vi "Update Crash Log.vi"(8 "New Crash Log Data":T1, 11 "Old Crash Log Data":T1) -> (3 "Updated Crash Log Data":T1)   [LabVIEW 2018, in "File IO.lvlib"]
doc: "Remove old data and add new data to the crash log."
uses:
  File IO.lvlib
  Top Level/Shared Controls/Analyzed Data Sets.ctl
  Top Level/Shared Controls/All Data Cluster.ctl
  Top Level/Shared Controls/Acq Data.ctl
  Top Level/Shared Controls/Post-Analysis Data.ctl
  Top Level/Shared Controls/Calculated Data.ctl
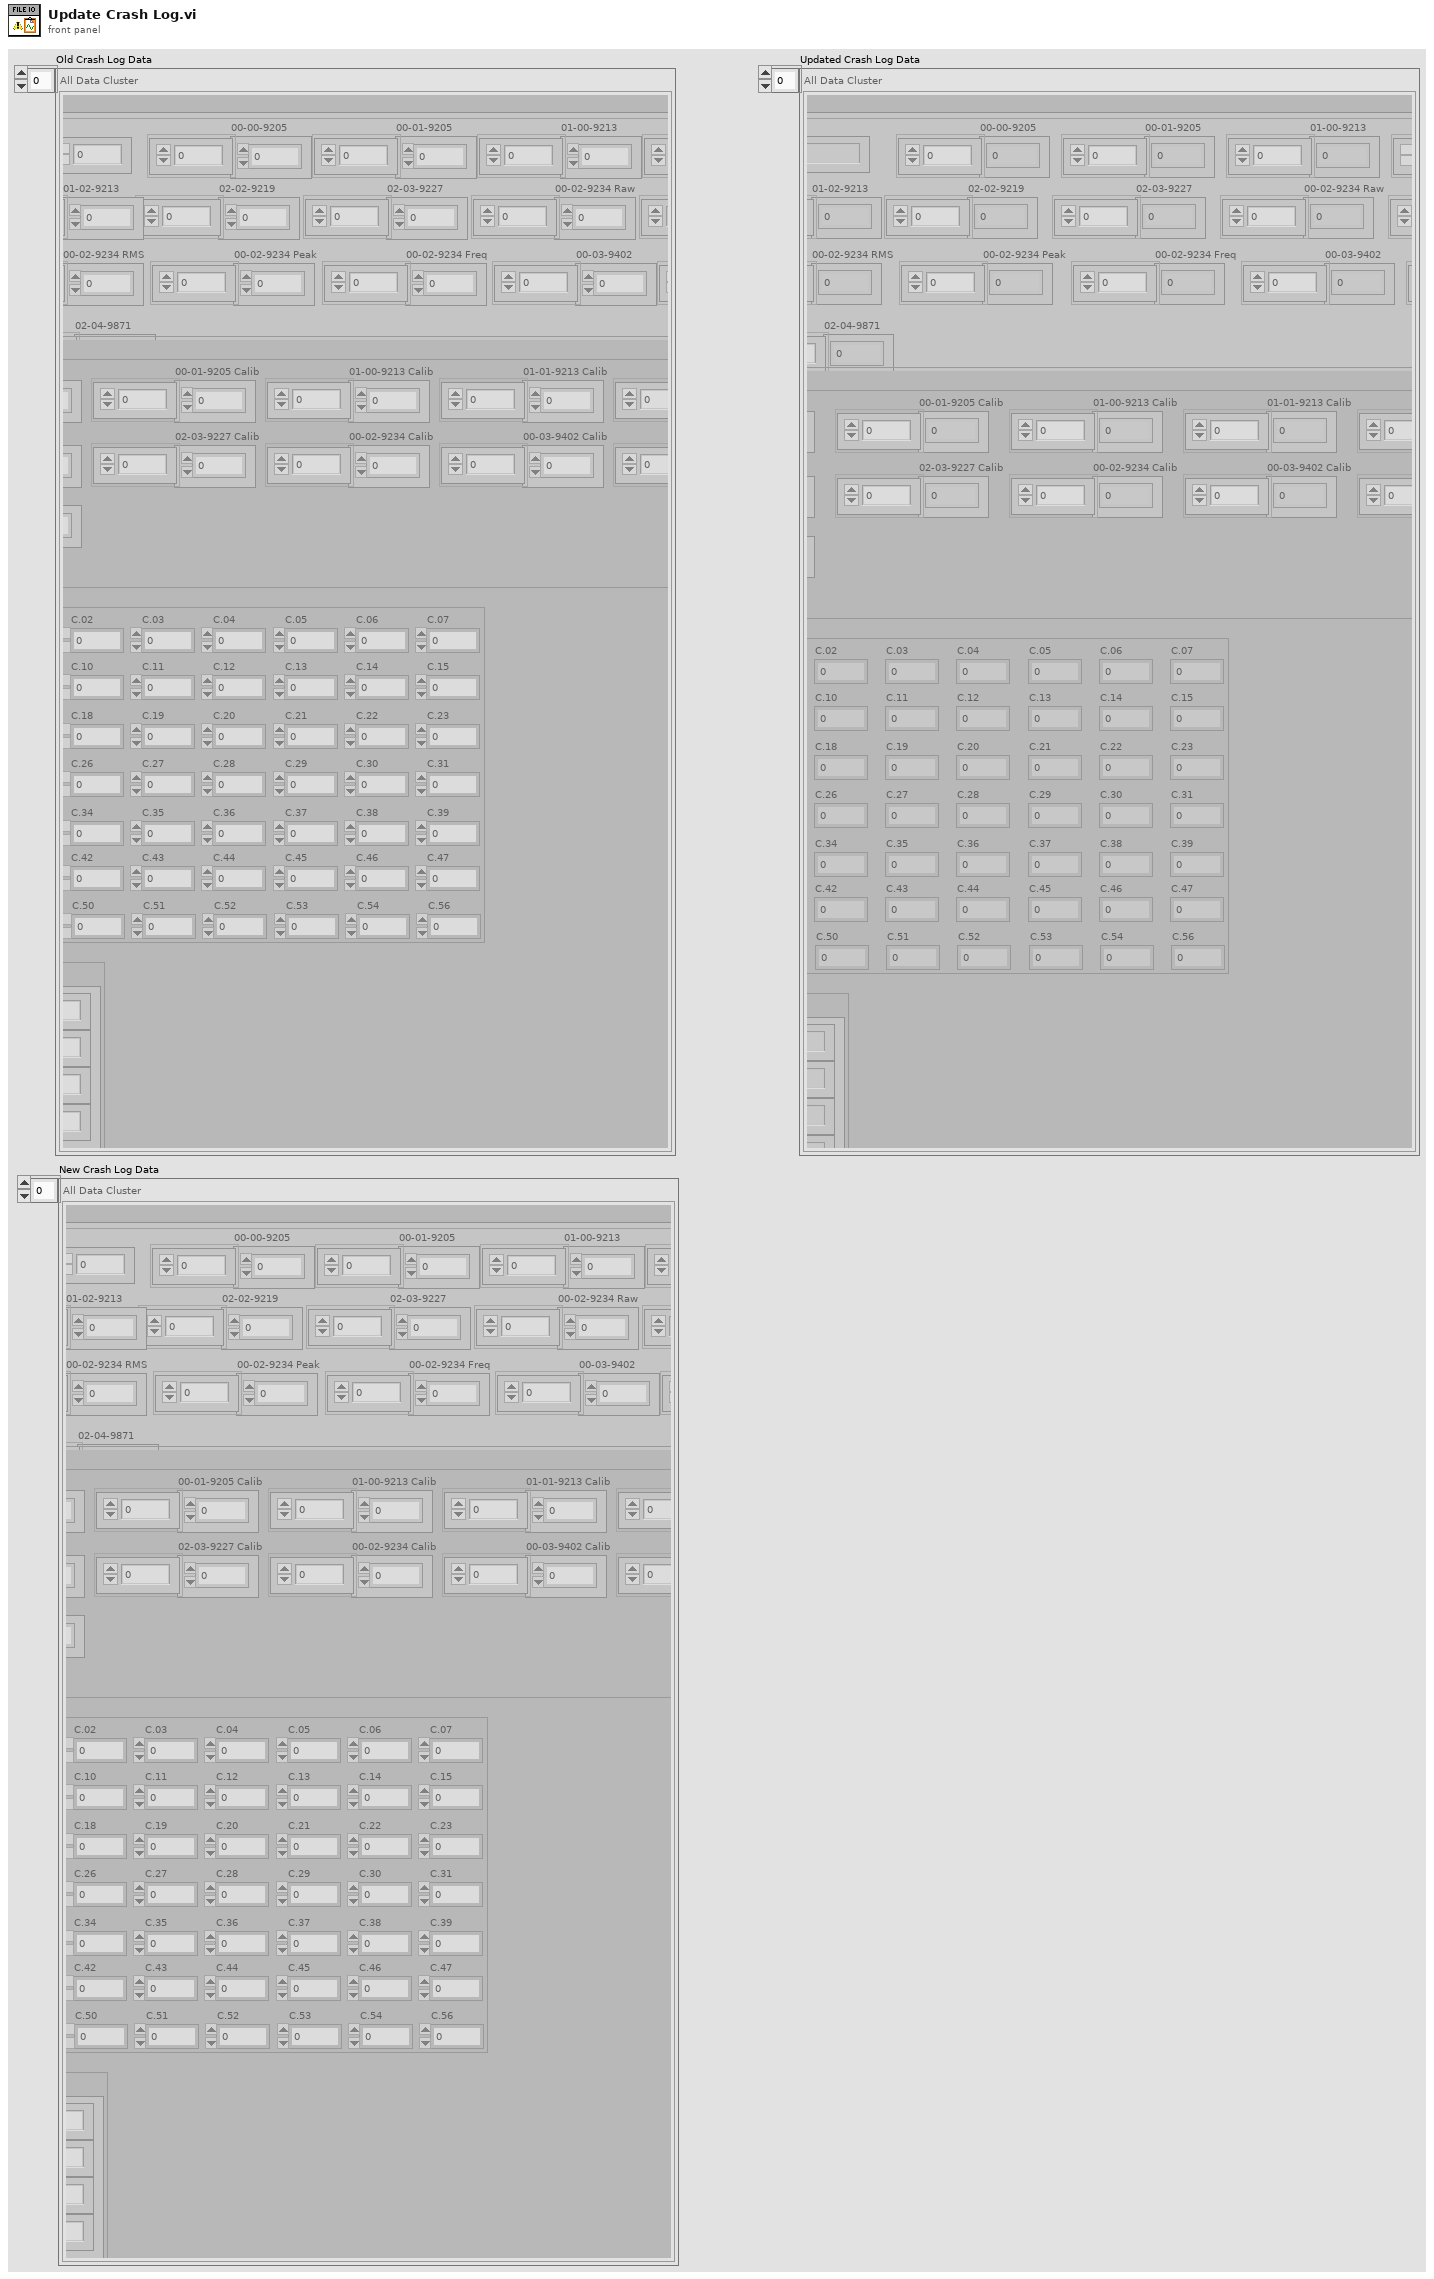
[diagram p1: front panel]
types:
  T1 = typedef "Analyzed Data Sets.ctl" = T2[]
  T2 = typedef "All Data Cluster.ctl" = cluster{"Acq Data":T3, "Post-Analysis Data":T4}
  T3 = typedef "Acq Data.ctl" = cluster{"Timestamp":timestamp, "Acq Period (ms)":i64, "00-00-9205":dbl[], "00-01-9205":dbl[], "01-00-9213":dbl[], "01-01-9213":dbl[], "01-02-9213":dbl[], "02-02-9219":dbl[], "02-03-9227":dbl[], "00-02-9234 Raw":dbl[], "00-02-9234 DC":dbl[], "00-02-9234 RMS":dbl[], "00-02-9234 Peak":dbl[], "00-02-9234 Freq":dbl[], "00-03-9402":dbl[], "02-05-9205":dbl[], "02-04-9871":dbl[]}
  T4 = typedef "Post-Analysis Data.ctl" = cluster{"Calibrated Data":cluster{"00-00-9205 Calib":dbl[], "00-01-9205 Calib":dbl[], "01-00-9213 Calib":dbl[], "01-01-9213 Calib":dbl[], "01-02-9213 Calib":dbl[], "02-02-9219 Calib":dbl[], "02-03-9227 Calib":dbl[], "00-02-9234 Calib":dbl[], "00-03-9402 Calib":dbl[], "02-05-9205 Calib":dbl[], "02-04-9871 2DArray":dbl[][]}, "Calculated Data":T5, "Indicator Data":cluster{"00-02-9234 Peak Vel (in/sec)":dbl[]}}
  T5 = typedef "Calculated Data.ctl" = cluster{"C.00":dbl, "C.01":dbl, "C.02":dbl, "C.03":dbl, "C.04":dbl, "C.05":dbl, "C.06":dbl, "C.07":dbl, "C.08":dbl, "C.09":dbl, "C.10":dbl, "C.11":dbl, "C.12":dbl, "C.13":dbl, "C.14":dbl, "C.15":dbl, "C.16":dbl, "C.17":dbl, "C.18":dbl, "C.19":dbl, "C.20":dbl, "C.21":dbl, "C.22":dbl, "C.23":dbl, "C.24":dbl, "C.25":dbl, "C.26":dbl, "C.27":dbl, "C.28":dbl, "C.29":dbl, "C.30":dbl, "C.31":dbl, "C.32":dbl, "C.33":dbl, "C.34":dbl, "C.35":dbl, "C.36":dbl, "C.37":dbl, "C.38":dbl, "C.39":dbl, "C.40":dbl, "C.41":dbl, "C.42":dbl, "C.43":dbl, "C.44":dbl, "C.45":dbl, "C.46":dbl, "C.47":dbl, "C.48":dbl, "C.49":dbl, "C.50":dbl, "C.51":dbl, "C.52":dbl, "C.53":dbl, "C.54":dbl, "C.56":dbl}
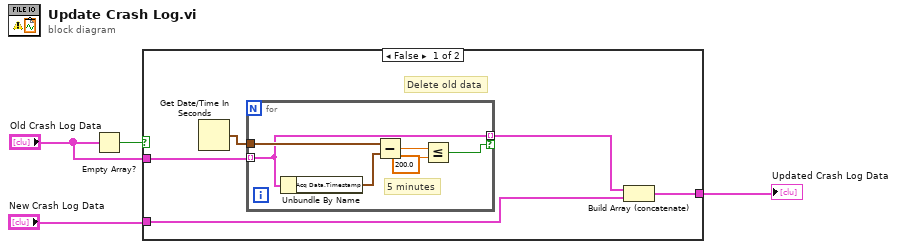
[diagram p0: block diagram]
diagram:
  n1 = Empty Array?(array="Old Crash Log Data") -> (empty?=w3:bool)
  n2 = case shown="False" w3 {
    tunnel: "New Crash Log Data" -> [w6 w16]
    tunnel: [w7 w16] -> w1
    tunnel: "Old Crash Log Data" -> [w9 _]
    frame False {
      # "Delete old data"
      n3 = Get Date/Time In Seconds() -> (seconds since 1Jan1904=w8:timestamp)
      n4 = for {
        tunnel: w9 -> [w11] mode=indexing
        tunnel: w8 -> [w12]
        tunnel: [w11] -> w5 mode=indexing if=w10
        # "5 minutes"
        n5 = Unbundle By Name(w11) -> ("Acq Data.Timestamp"=w15:timestamp)
        n6 = Subtract(x=w12, y=w15) -> (x-y=w14:dbl)
        n7 = Less Or Equal?(x=w14, y=200.0) -> (x <= y?=w10:bool)
      }
      n8 = Build Array (concatenate)(w5, w6) -> (w7:T1)
    }
    frame True {
    }
  }
  "Updated Crash Log Data" <- w1
